vi "rad_Configure Targets Settings Dialog.vi"(11 "Targets Settings":T1) -> (1 "Cancelled":bool, 3 "Targets Settings":T1)   [LabVIEW 2021]
uses:
  TypeDefs/rad_Targets Settings.ctl
  Util/FP Control/FP Control Functions.ctl
  rad_Globals.vi
panel:
  in  "Global Timeout (ms)":u32=4000
  in  "Reduce Discovery\nTimeout":bool
  in  "Other":bool
  in  "User Targets Only":bool
  in  "PXI":bool
  in  "FP":bool
  in  "cRIO":bool
  in  "Cancel":bool
  in  "OK":bool
  # "Targets to Display"
  # "Target Types"
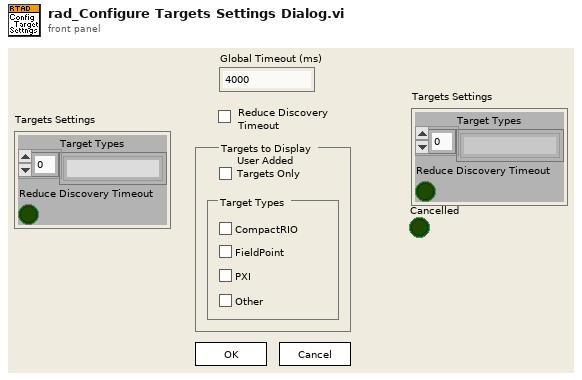
[diagram p1: front panel]
types:
  T1 = typedef "rad_Targets Settings.ctl" = cluster{"Target Types":string[], "Reduce Discovery Timeout":bool}
  T2 = typedef "FP Control Functions.ctl" = enum16{"Open", "Close", "Bring To Front", "Center"}
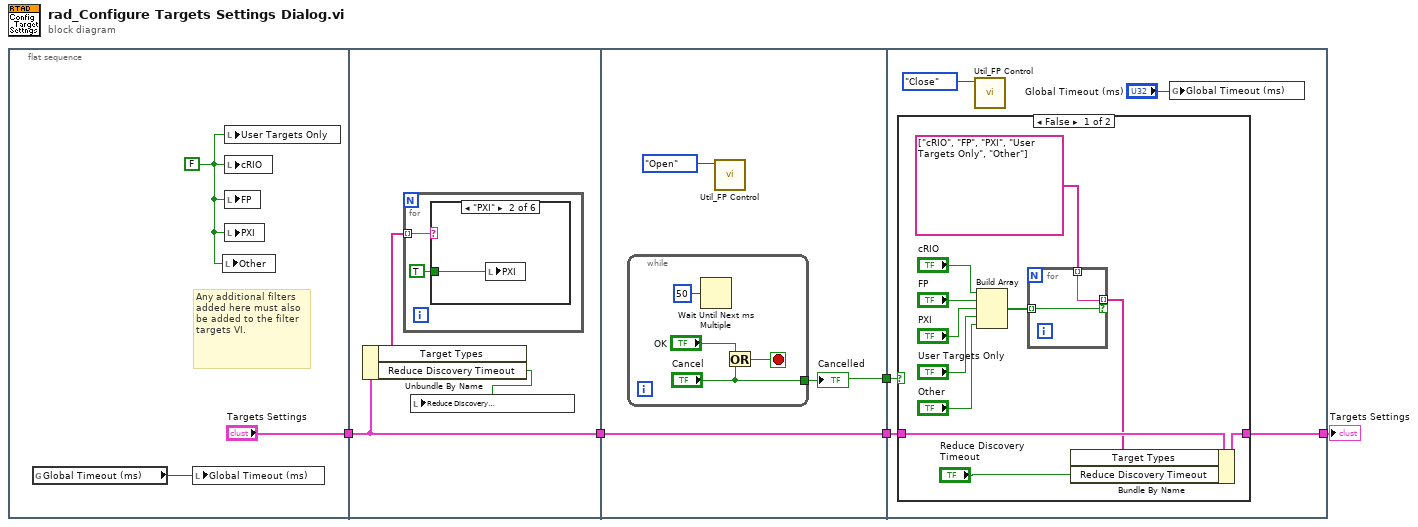
[diagram p0: block diagram]
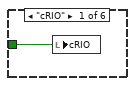
[diagram p2: hidden frame]
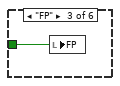
[diagram p3: hidden frame]
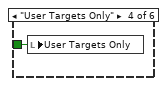
[diagram p4: hidden frame]
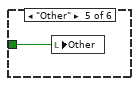
[diagram p5: hidden frame]
diagram:
  n1 = flat-sequence {
    tunnel: ["Targets Settings"] -> w1
    tunnel: [w11] -> w2
    tunnel: w1 -> [w11]
    tunnel: [w21] -> w5
    tunnel: [w20] -> w4
    tunnel: w2 -> [w20]
    tunnel: w5 -> [w30]
    tunnel: w4 -> [w29]
    tunnel: [w28] -> w3
    frame #0 {
      w7 = FALSE
      # "Any additional filters added here must also be added to the filter targets VI."
      n2 = global read "rad_Globals.vi" "Global Timeout (ms)"() -> (w6:u32)
      n3 = local write "Global Timeout (ms)"(w6) -> ()
      n4 = local write "Other"(w7) -> ()
      n5 = local write "User Targets Only"(w7) -> ()
      n6 = local write "cRIO"(w7) -> ()
      n7 = local write "FP"(w7) -> ()
      n8 = local write "PXI"(w7) -> ()
    }
    frame #1 {
      n9 = Unbundle By Name(w11) -> ("Target Types"=w10:string[], "Reduce Discovery Timeout"=w9:bool)
      n10 = for {
        tunnel: w10 -> [w13] mode=indexing
        n11 = case shown="\"PXI\"" w13 {
          tunnel: TRUE -> [w14 w15 w16 w17 w18 _]
          frame "cRIO" {
            n12 = local write "cRIO"(w14) -> ()
          }
          frame "PXI" {
            n13 = local write "PXI"(w15) -> ()
          }
          frame "FP" {
            n14 = local write "FP"(w16) -> ()
          }
          frame "User Targets Only" {
            n15 = local write "User Targets Only"(w17) -> ()
          }
          frame "Other" {
            n16 = local write "Other"(w18) -> ()
          }
          frame Default {
          }
        }
      }
      n17 = local write "Reduce Discovery\nTimeout"(w9) -> ()
    }
    frame #2 {
      n18 = while {
        tunnel: ["Cancel"] -> w21
        stop <- w23 stop-if-true
        n19 = Wait Until Next ms Multiple(millisecond multiple=u32 50) -> ()  [unwired: 1 out]
        n20 = Or(x="OK", y="Cancel") -> (x .or. y?=w23:bool)
      }
      "Cancelled" <- w21
      n21 = call "Util_FP Control.vi"("Function"=FP_Control_Functions."Open") -> ()  [unwired: 1 in, 10 out]
    }
    frame #3 {
      n22 = case shown="False" w30 {
        tunnel: w29 -> [w36 w44]
        tunnel: [w35 w44] -> w28
        frame False {
          n23 = Build Array("cRIO", "FP", "PXI", "User Targets Only", "Other") -> (w38:bool[])
          n24 = for {
            tunnel: w38 -> [w42] mode=indexing
            tunnel: string[] ["cRIO", "FP", "PXI", "User Targets Only", "Other"] -> [w43] mode=indexing
            tunnel: [w43] -> w31 mode=indexing if=w42
          }
          n25 = Bundle By Name(cluster=w36, "Target Types"=w31, "Reduce Discovery Timeout"="Reduce Discovery\nTimeout") -> (w35:T1)
        }
        frame True {
        }
      }
      n26 = call "Util_FP Control.vi"("Function"=FP_Control_Functions."Close") -> ()  [unwired: 1 in, 10 out]
      n27 = global write "rad_Globals.vi" "Global Timeout (ms)"("Global Timeout (ms)") -> ()
    }
  }
  "Targets Settings" <- w3
